vi "Is Call Cancelled.vi"(8 "error in":errorcluster, 11 "gRPCid in":T1) -> (0 "error out":errorcluster, 2 "Is Cancelled":bool, 3 "gRPCid out":T1)   [LabVIEW 2019, in "grpc-lvsupport.lvlib"]
uses:
  grpc-lvsupport.lvlib
  grpcId.ctl
  <resource>/labview_grpc_server.dll
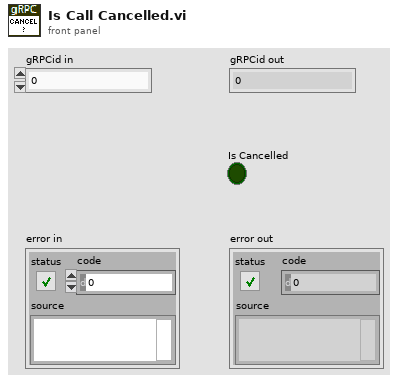
[diagram p1: front panel]
types:
  T1 = typedef "grpc-lvsupport.lvlib/grpcId.ctl" = u64
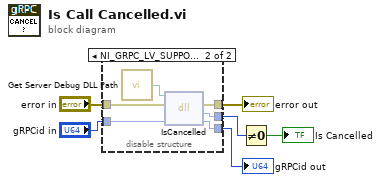
[diagram p0: block diagram]
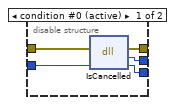
[diagram p2: hidden frame]
diagram:
  n1 = disable-structure shown="NI_GRPC_LV_SUPPORT_DEBUG==True&&RUN_TIME_ENGINE==False" {
    disable-tunnel: [w11 w17] -> w6
    disable-tunnel: "error in" -> [w10 w16]
    disable-tunnel: "gRPCid in" -> [w9 w15]
    disable-tunnel: [w8 w14] -> w3
    disable-tunnel: [w7 w13] -> w2
    frame condition #0 (active) {
      n2 = dll-call lib="C:/Program Files (x86)/National Instruments/LabVIEW 2024/resource/labview_grpc_server.*" fn="IsCancelled"(error in=w10, "id"=w9) -> (error out=w11:errorcluster, "return type"=w7:i32, "id"=w8:T1)  [unwired: 2 in, 1 out]
    }
    frame condition #1 {
      n3 = call "Get Server Debug DLL Path.vi"() -> ("DLL Path"=w12:path)
      n4 = dll-call lib="?" fn="IsCancelled"(path in=w12, error in=w16, "id"=w15) -> (error out=w17:errorcluster, "return type"=w13:i32, "id"=w14:T1)  [unwired: 1 in, 1 out]
    }
  }
  "gRPCid out" <- w3
  "error out" <- w6
  n5 = Not Equal To 0?(x=w2) -> (x != 0?=→"Is Cancelled":bool)
